vi "CreateSocketHandler.vi"(7 "Port":i32, 8 "error in (no error)":errorcluster, 10 "Address (127.0.0.1)":string="127.0.0.1", 11 "Logger in":refnum<class "Logger.lvclass">) -> (0 "error out":errorcluster, 2 "SocketHandler":refnum<class "SocketHandler.lvclass">, 3 "Logger out":refnum<class "Logger.lvclass">)   [LabVIEW 2022 SP3, in "Logger.lvlib" / "Logger.lvclass"]
uses:
  Logger.lvclass
  C:/Users/jakub/repos/gh/PythonWrapper/Source/PythonWrapper/PythonWrapper.lvclass
  SocketHandler/SocketHandler.lvclass
  C:/Users/jakub/repos/gh/Logger/Source/Handler/Handler.lvclass
  PythonWrapper/Source/PythonWrapper/PythonWrapper.lvclass/PythonWrapper.ctl
  Logger.lvclass/Logger.ctl
  Handler/Handler.lvclass/Handler.ctl
  PythonWrapper/Source/PythonWrapper/Read PythonSession.vi
  PythonWrapper/Source/PythonWrapper/Read ModulePath.vi
  Read FunctionCreateFileHandler.vi
  Read Logger.vi
  Handler/Write Name.vi
  Handler/Write Handler.vi
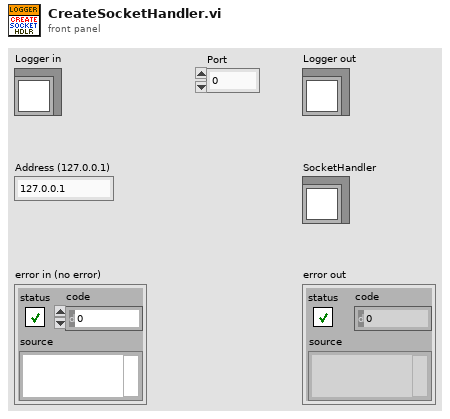
[diagram p1: front panel]
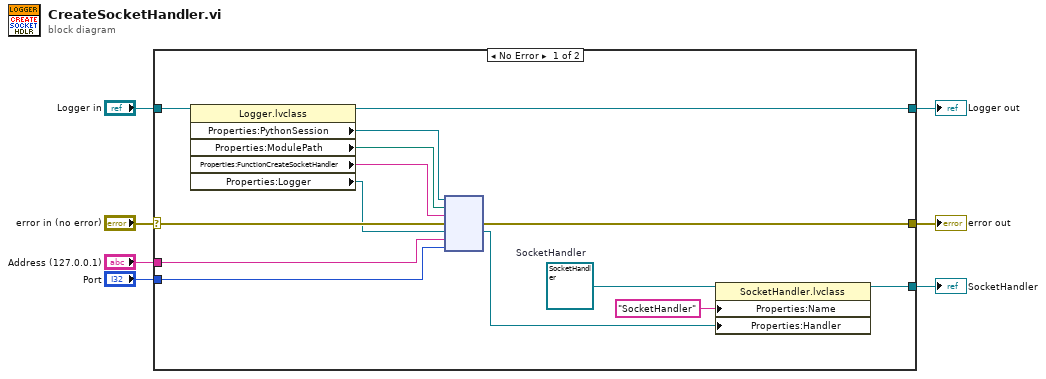
[diagram p0: block diagram]
diagram:
  n1 = case shown="No Error" "error in (no error)" {
    selector: "error in (no error)" -> [w19 w23]
    tunnel: [w12 w23] -> w4
    tunnel: [w20 w22] -> w6
    tunnel: "Logger in" -> [w21 w22]
    tunnel: "Address (127.0.0.1)" -> [w14 _]
    tunnel: "Port" -> [w13 _]
    tunnel: [w8 _] -> w3
    frame No Error {
      w11 = refnum<class "SocketHandler.lvclass"> refnum  # SocketHandler
      n2 = property class="Logger.lvclass"(reference=w21) -> (reference out=w20:refnum<class "Logger.lvclass">, "Properties:PythonSession"=w18:refnum<k35>, "Properties:ModulePath"=w16:path, "Properties:FunctionCreateSocketHandler"=w17:string, "Properties:Logger"=w15:refnum<k38>)  [unwired: 1 in, 1 out]
      n3 = node(w18, w16, w17, w19, w15, w14, w13) -> (w12:errorcluster, w9:refnum<k38>)  [unwired: 2 in, 3 out]
      n4 = property class="SocketHandler.lvclass"(reference=w11, "Properties:Name"="SocketHandler" ("Name"), "Properties:Handler"=w9) -> (reference out=w8:refnum<class "SocketHandler.lvclass">)  [unwired: 1 in, 1 out]
    }
    frame Error {
    }
  }
  "error out" <- w4
  "Logger out" <- w6
  "SocketHandler" <- w3
